vi "GetGraphAppearance(SubVI).vi"(8 "Error In":errorcluster, 9 "Str Refnum":refnum<vi>, 10 "Enum Refnum":refnum<vi>, 11 "Cluster in":refnum<vi>) -> (0 "Error Out":errorcluster)   [LabVIEW 2018]
uses:
  CTL/Graph settings.ctl
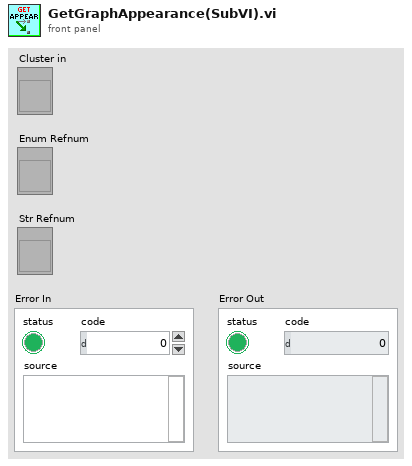
[diagram p1: front panel]
types:
  T1 = typedef "Graph settings.ctl" = cluster{"Axis X Min":dbl, "Axis X Name":string, "Axis X Max":dbl, "Axis Y Min":dbl, " Axis Y Name":string, "Axis Y Max":dbl, "Autoscale":enum16{"Yes", "No", "Only Oy", "Only Ox"}, "Choice Line":dbl}
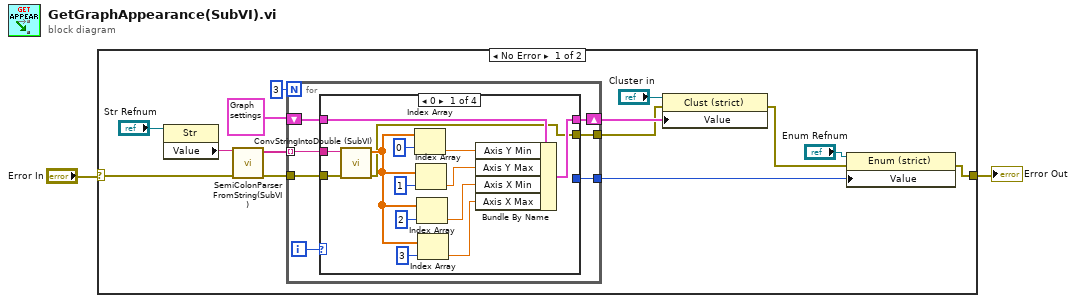
[diagram p0: block diagram]
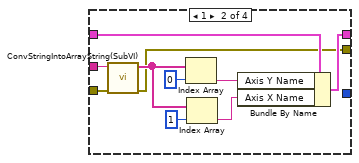
[diagram p2: hidden frame]
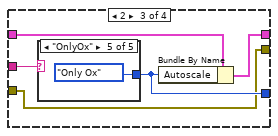
[diagram p3: hidden frame]
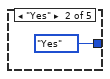
[diagram p5: hidden frame]
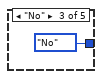
[diagram p6: hidden frame]
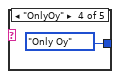
[diagram p7: hidden frame]
diagram:
  n1 = case shown="No Error" "Error In" {
    selector: "Error In" -> [w6 w58]
    tunnel: [w4 w58] -> w1
    frame No Error {
      n2 = property on="Property Node" class="Str"(reference="Str Refnum") -> ("Value"=w15:string)  [unwired: 1 in, 2 out]
      n3 = call "SemiColonParserFromString(SubVI).vi"("Error In"=w6, "String In"=w15) -> ("Error Out"=w7:errorcluster, "String Array Out"=w16:string[])  [unwired: 8 in]
      n4 = for {
        N: 3 -> [_]
        tunnel: w16 -> [w22] mode=indexing
        shift-right: [w21] -> w12
        shift-left: T1 {"Axis X Min"=0.0, "Axis X Name"="", "Axis X Max"=1.0, "Axis Y Min"=0.0, " Axis Y Name"="", "Axis Y Max"=1.0, "Autoscale"=enum."Yes", "Choice Line"=0.0} ("Value") -> [w20]
        tunnel: [w19] -> w11
        tunnel: w7 -> [w18]
        tunnel: [w17] -> w3
        i -> [w23]
        n5 = case shown="0" w23 {
          tunnel: w22 -> [w32 w44 w52 _]
          tunnel: [w26 w40 w50 _] -> w21
          tunnel: w20 -> [w27 w41 w51 _]
          tunnel: [_ _ w49 _] -> w19
          tunnel: w18 -> [w25 w39 w48 w57]
          tunnel: [w24 w38 w48 w57] -> w17
          frame 0 {
            n6 = call "ConvStringIntoDouble (SubVI).vi"("Error In"=w25, "String In"=w32) -> ("Error Out"=w24:errorcluster, "Array Out"=w37:dbl[])  [unwired: 6 in]
            n7 = Index Array(array=w37, index=0) -> (element=w31:dbl)
            n8 = Index Array(array=w37, index=1) -> (element=w30:dbl)
            n9 = Index Array(array=w37, index=2) -> (element=w29:dbl)
            n10 = Index Array(array=w37, index=3) -> (element=w28:dbl)
            n11 = Bundle By Name(cluster=w27, "Axis Y Min"=w31, "Axis Y Max"=w30, "Axis X Min"=w29, "Axis X Max"=w28) -> (w26:T1)
          }
          frame 1 {
            n12 = call "ConvStringIntoArrayString(SubVI).vi"("Error In"=w39, "String In"=w44) -> ("Error Out"=w38:errorcluster, "Array String Out"=w47:string[])  [unwired: 8 in]
            n13 = Index Array(array=w47, index=0) -> (element=w43:string)
            n14 = Index Array(array=w47, index=1) -> (element=w42:string)
            n15 = Bundle By Name(cluster=w41, "Axis Y Name"=w43, "Axis X Name"=w42) -> (w40:T1)
          }
          frame 2 {
            n16 = case shown="\"OnlyOx\"" w52 {
              tunnel: [_ enum16{"Yes", "No", "Only Oy", "Only Ox"}."Yes" ("Value") enum16{"Yes", "No", "Only Oy", "Only Ox"}."No" ("Value") enum16{"Yes", "No", "Only Oy", "Only Ox"}."Only Oy" ("Value") enum16{"Yes", "No", "Only Oy", "Only Ox"}."Only Ox" ("Value")] -> w49
              frame "False", Default {
              }
              frame "Yes" {
              }
              frame "No" {
              }
              frame "OnlyOy" {
              }
              frame "OnlyOx" {
              }
            }
            n17 = Bundle By Name(cluster=w51, "Autoscale"=w49) -> (w50:T1)
          }
          frame Default {
          }
        }
      }
      n18 = property on="Property Node" class="Clust (strict)"(reference="Cluster in", error in=w3, "Value"=w12) -> (error out=w5:errorcluster)  [unwired: 1 out]
      n19 = property on="Property Node" class="Enum (strict)"(reference="Enum Refnum", error in=w5, "Value"=w11) -> (error out=w4:errorcluster)  [unwired: 1 out]
    }
    frame Error {
    }
  }
  "Error Out" <- w1
